vi "NotifyUIHidden.vi"(8 "error in (no error)":errorcluster, 11 "SMO.UI":refnum<class "SMO.UI.lvclass">) -> (0 "error out":errorcluster, 3 "SMO.UI out":refnum<class "SMO.UI.lvclass">)   [LabVIEW 2021, in "smo.lvlib" / "SMO.UI.lvclass"]
uses:
  SMO.UI.lvclass
  SMO.UI.lvclass/SMO.UI.ctl
  SMO.UI.ReftoDVR.vi
panel:
  # "For instructions on how to use the JKI State Machine Objects, examples and video tutorials, visit:\nhttp://jki.net/state-machine-objects/\n\nJKI State Machine Objects™\nhttp://jki.net/state-machine-objects/\nCopyright (C) 2005-2015, JKI <info@jki.net>\nALL RIGHTS RESERVED"
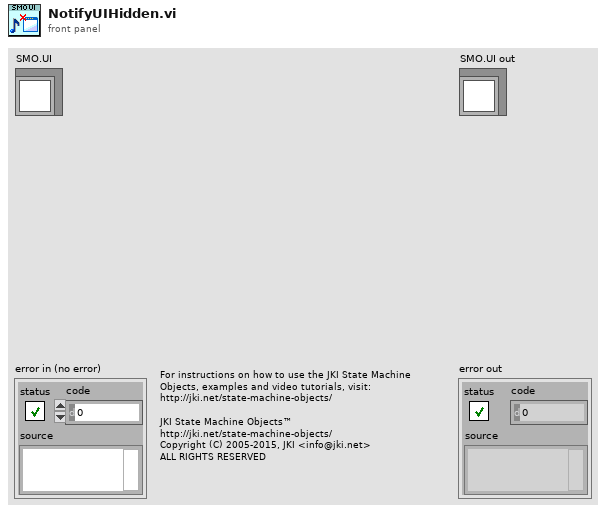
[diagram p1: front panel]
types:
  T1 = typedef "smo.lvlib/SMO.UI.lvclass/PublicEvents--Cluster.ctl" = cluster{"UI Hidden":refnum<user-event>, "UI State":refnum<user-event>}
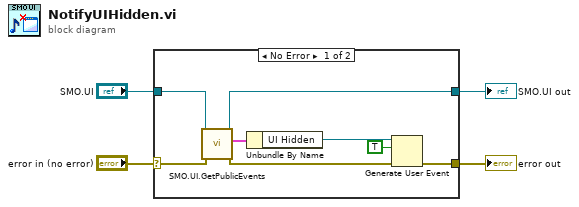
[diagram p0: block diagram]
diagram:
  n1 = case shown="No Error" "error in (no error)" {
    selector: "error in (no error)" -> [w10 w14]
    tunnel: [w5 w14] -> w3
    tunnel: [w11 w13] -> w1
    tunnel: "SMO.UI" -> [w12 w13]
    frame No Error {
      n2 = call "SMO.UI.GetPublicEvents.vi"("error in (no error)"=w10, "SMO.UI"=w12) -> ("error out"=w6:errorcluster, "SMO.UI Public Events"=w9:T1, "SMO.UI out"=w11:refnum<class "SMO.UI.lvclass">)  [unwired: 7 in]
      n3 = Unbundle By Name(w9) -> ("UI Hidden"=w8:refnum<user-event>)
      n4 = Generate User Event(user event=w8, event data cluster=TRUE ("event data"), error in=w6) -> (error out=w5:errorcluster)  [unwired: 1 in, 1 out]
    }
    frame Error {
    }
  }
  "error out" <- w3
  "SMO.UI out" <- w1
